vi "Ramp.vi"(0 "VISA resource name":refnum<visa-resource-name>, 11 "error in (no error)":errorcluster) -> (4 "VISA resource name out":refnum<visa-resource-name>, 6 "Ramping On/Off":bool, 8 "Rate Value (0.001)":dbl=0.001 min=0.001 max=10.0 step=0.001 format="%.3f", 10 "Ramping Active/Inactive":bool, 15 "error out":errorcluster)   [LabVIEW 2021, in "Lake Shore Cryotronics 370.lvlib"]
doc: "This VI displays the parameters of the ramp function."
uses:
  Lake Shore Cryotronics 370.lvlib
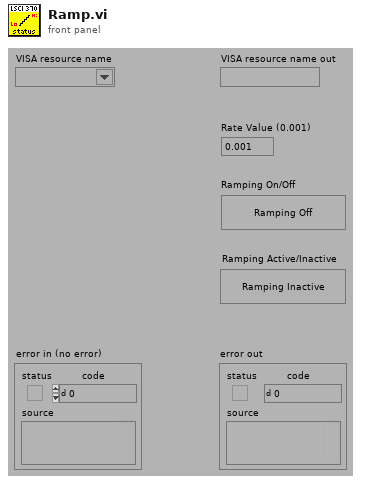
[diagram p1: front panel]
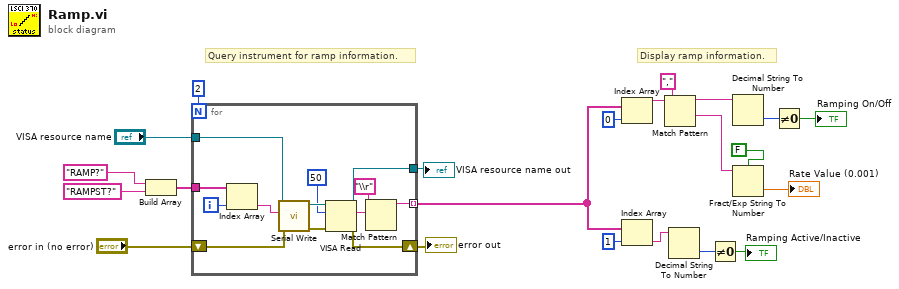
[diagram p0: block diagram]
diagram:
  # "Display ramp information."
  # "Query instrument for ramp information."
  n1 = Build Array("RAMP?", "RAMPST?") -> (w18:string[])
  n2 = for {
    N: 2 -> [_]
    tunnel: w18 -> [w31]
    shift-right: [w28] -> w21
    shift-left: "error in (no error)" -> [w29]
    tunnel: [w27] -> w22
    tunnel: [w25] -> w3 mode=indexing
    tunnel: "VISA resource name" -> [w24]
    i -> [w30]
    n3 = Index Array(array=w31, index=w30) -> (element=w23:string)
    n4 = call "Serial Write.vi"("error in (no error)"=w29, "Write Buffer (\"\")"=w23, "VISA resource name"=w24) -> ("error out"=w34:errorcluster, "VISA resource name out"=w35:refnum<visa-resource-name>)  [unwired: 6 in, 1 out]
    n5 = VISA Read(VISA resource name=w35, byte count=50, error in (no error)=w34) -> (VISA resource name out=w27:refnum<visa-resource-name>, read buffer=w32:string, error out=w28:errorcluster)  [unwired: 1 out]
    n6 = Match Pattern(string=w32, regular expression="\\r") -> (before substring=w25:string)  [unwired: 1 in, 3 out]
  }
  "VISA resource name out" <- w22
  "error out" <- w21
  n7 = Index Array(array=w3, index=0) -> (element=w12:string)
  n8 = Index Array(array=w3, index=1) -> (element=w5:string)
  n9 = Match Pattern(string=w12, regular expression=",") -> (before substring=w11:string, after substring=w8:string)  [unwired: 1 in, 2 out]
  n10 = Decimal String To Number(string=w5) -> (number=w6:i32)  [unwired: 2 in, 1 out]
  n11 = Not Equal To 0?(x=w6) -> (x != 0?=→"Ramping Active/Inactive":bool)
  n12 = Decimal String To Number(string=w11) -> (number=w10:i32)  [unwired: 2 in, 1 out]
  n13 = Fract/Exp String To Number(use system decimal point (T)=FALSE, string=w8) -> (number=→"Rate Value (0.001)":dbl)  [unwired: 2 in, 1 out]
  n14 = Not Equal To 0?(x=w10) -> (x != 0?=→"Ramping On/Off":bool)
